vi "Roughness_filenamer.vi"() -> (0 "String":string)   [LabVIEW 2010]
uses:
  Results_plotter_Global.vi
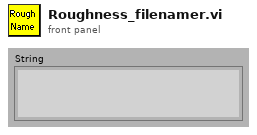
[diagram p1: front panel]
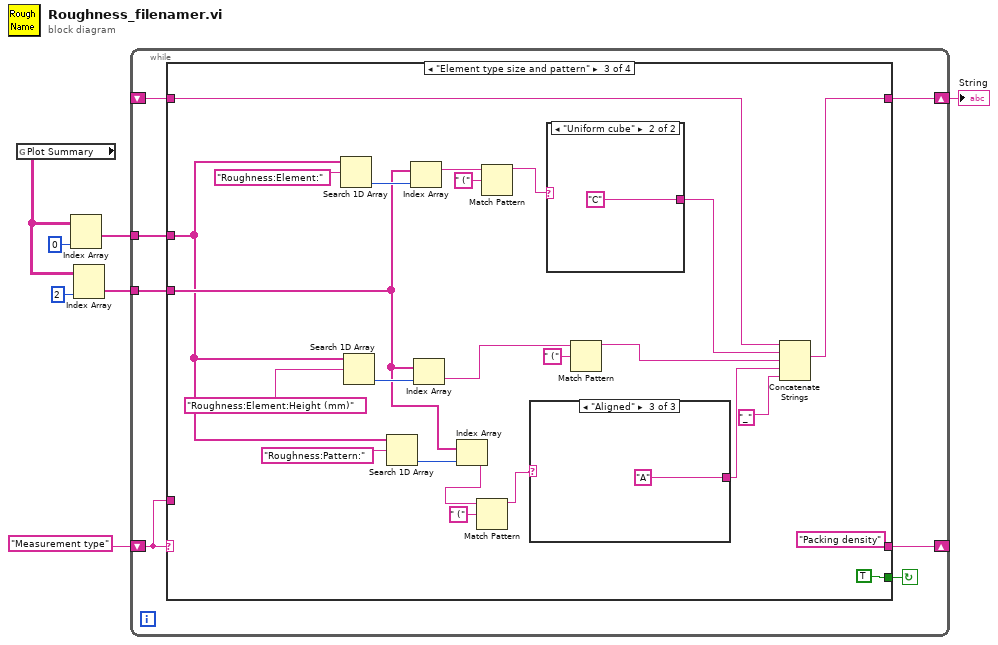
[diagram p0: block diagram]
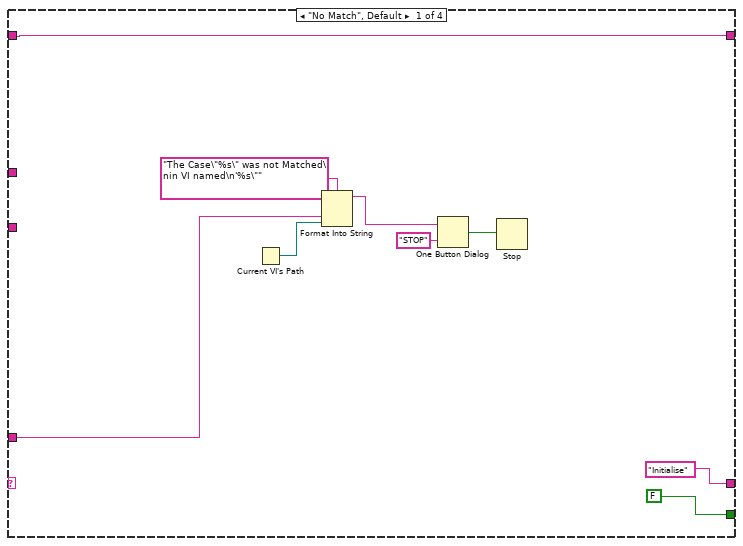
[diagram p2: hidden frame]
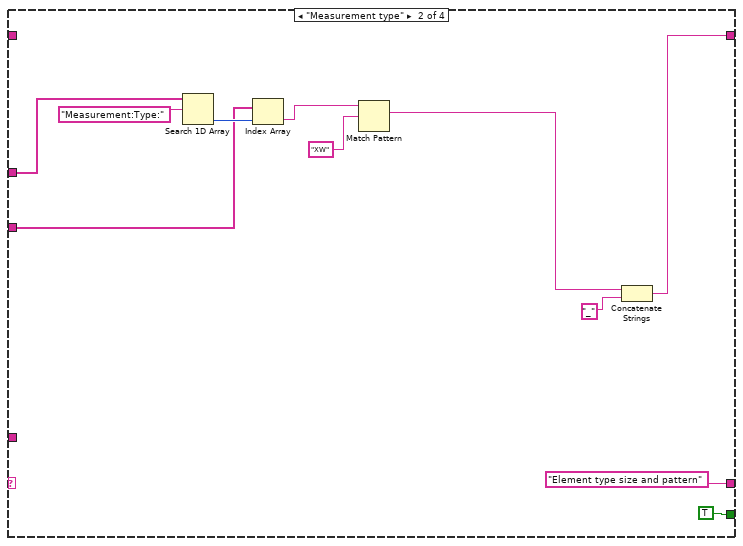
[diagram p3: hidden frame]
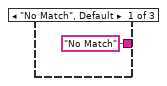
[diagram p4: hidden frame]
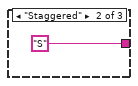
[diagram p5: hidden frame]
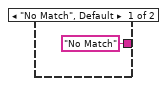
[diagram p6: hidden frame]
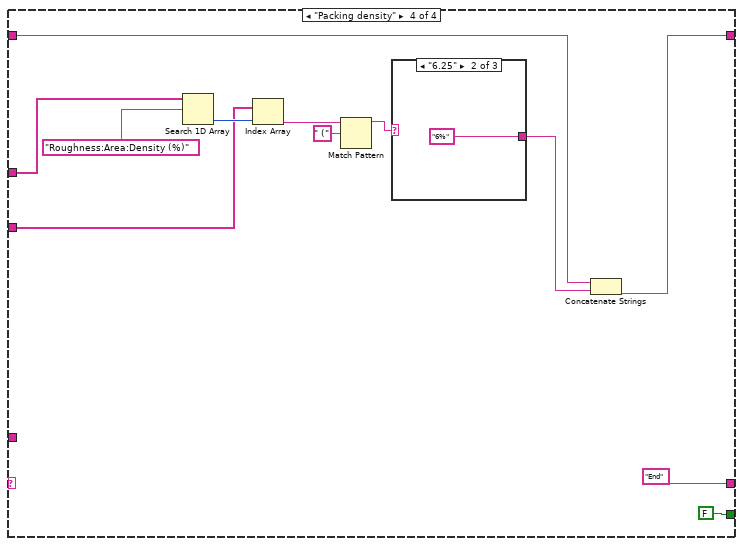
[diagram p7: hidden frame]
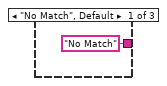
[diagram p8: hidden frame]
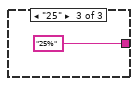
[diagram p9: hidden frame]
diagram:
  n1 = global read "Results_plotter_Global.vi" "Plot Summary"() -> (w4:string[][])
  n2 = Index Array(array=w4, index (col)=0 ("disabled index (col)")) -> (element=w3:string[])  [unwired: 1 in]
  n3 = Index Array(array=w4, index (col)=2 ("disabled index (col)")) -> (element=w2:string[])  [unwired: 1 in]
  n4 = while {
    shift-left: "Measurement type" -> [w12]
    shift-right: [w13] -> _
    tunnel: w3 -> [w11]
    tunnel: w2 -> [w10]
    shift-right: [w9] -> w1
    shift-left: _ -> [w8]
    stop <- w14 continue-if-true
    n5 = case shown="\"Element type size and pattern\"" w12 {
      tunnel: [FALSE TRUE TRUE FALSE] -> w14
      tunnel: ["Initialise" "Element type size and pattern" "Packing density" "End"] -> w13
      tunnel: w12 -> [w18 _ _ _]
      tunnel: w11 -> [_ w26 w47 w71]
      tunnel: w10 -> [_ w25 w48 w67]
      tunnel: [w15 w30 w51 w69] -> w9
      tunnel: w8 -> [w15 _ w44 w68]
      frame "No Match", Default {
        n6 = Current VI's Path() -> (path=w17:path)
        n7 = Format Into String(format string="The Case\"%s\" was not Matched\nin VI named\n'%s\"" ("Format String"), w18, w17) -> (resulting string=w21:string)  [unwired: 2 in, 1 out]
        n8 = One Button Dialog(message=w21, button name ("OK")="STOP") -> (true=w19:bool)
        n9 = Stop(stop? (T)=w19) -> ()
      }
      frame "Measurement type" {
        n10 = Search 1D Array(1D array=w26, element="Measurement:Type:") -> (index of element=w32:i32)  [unwired: 1 in]
        n11 = Index Array(array=w25, index=w32) -> (element=w28:string)
        n12 = Match Pattern(string=w28, regular expression="XW") -> (match substring=w27:string)  [unwired: 1 in, 3 out]
        n13 = Concatenate Strings(w27, "_") -> (w30:string)
      }
      frame "Element type size and pattern" {
        n14 = Search 1D Array(1D array=w47, element="Roughness:Element:") -> (index of element=w56:i32)  [unwired: 1 in]
        n15 = Search 1D Array(1D array=w47, element="Roughness:Element:Height (mm)") -> (index of element=w53:i32)  [unwired: 1 in]
        n16 = Search 1D Array(1D array=w47, element="Roughness:Pattern:") -> (index of element=w49:i32)  [unwired: 1 in]
        n17 = Index Array(array=w48, index=w56) -> (element=w43:string)
        n18 = Index Array(array=w48, index=w53) -> (element=w39:string)
        n19 = Index Array(array=w48, index=w49) -> (element=w36:string)
        n20 = Match Pattern(string=w36, regular expression=" (") -> (before substring=w35:string)  [unwired: 1 in, 3 out]
        n21 = Match Pattern(string=w43, regular expression=" (") -> (before substring=w41:string)  [unwired: 1 in, 3 out]
        n22 = case shown="\"Aligned\"" w35 {
          tunnel: ["No Match" "S" "A"] -> w46
          frame "No Match", Default {
          }
          frame "Staggered" {
          }
          frame "Aligned" {
          }
        }
        n23 = case shown="\"Uniform cube\"" w41 {
          tunnel: ["No Match" "C"] -> w52
          frame "No Match", Default {
          }
          frame "Uniform cube" {
          }
        }
        n24 = Match Pattern(string=w39, regular expression=" (") -> (before substring=w38:string)  [unwired: 1 in, 3 out]
        n25 = Concatenate Strings(w44, w52, w38, w46, "_") -> (w51:string)
      }
      frame "Packing density" {
        n26 = Search 1D Array(1D array=w71, element="Roughness:Area:Density (%)") -> (index of element=w73:i32)  [unwired: 1 in]
        n27 = Index Array(array=w67, index=w73) -> (element=w65:string)
        n28 = Match Pattern(string=w65, regular expression=" (") -> (before substring=w64:string)  [unwired: 1 in, 3 out]
        n29 = case shown="\"6.25\"" w64 {
          tunnel: ["No Match" "6%" "25%"] -> w70
          frame "No Match", Default {
          }
          frame "6.25" {
          }
          frame "25" {
          }
        }
        n30 = Concatenate Strings(w68, w70) -> (w69:string)
      }
    }
  }
  "String" <- w1
